vi "Broadcast Status.vi"(8 "error in (no error)":errorcluster, 11 "Actor in":refnum<class "System Status Actor.lvclass">) -> (0 "error out":errorcluster)   [LabVIEW 2020, in "System Status Actor.lvclass"]
uses:
  System Status Actor.lvclass
  System Status Actor.lvclass/System Status Actor.ctl
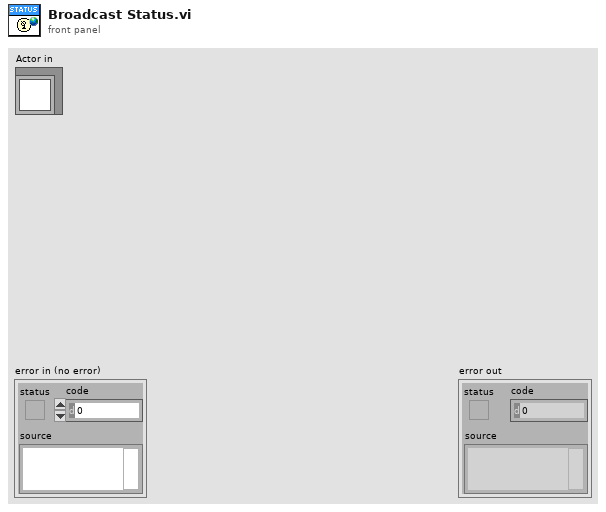
[diagram p1: front panel]
types:
  T1 = typedef "System Status Actor.lvclass/Status.ctl" = cluster{"Memory":cluster{"Total [MB]":dbl, "Used [MB]":dbl, "Free [MB]":dbl}, "Disk":cluster{"Total [MB]":dbl, "Used [MB]":dbl, "Free [MB]":dbl}, "CPU loads":T2[]}
  T2 = typedef "NI_Real-Time Target Support.lvlib/RT CPU Load.ctl" = cluster{"Total (%)":dbl, "Time Critical (%)":dbl, "Timed Structures (%)":dbl, "High (%)":dbl, "Above Normal (%)":dbl, "Normal (%)":dbl, "Background (%)":dbl, "Idle (%)":dbl, "ISR (%)":dbl}
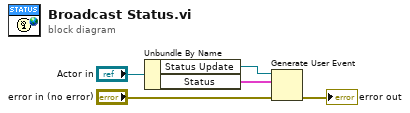
[diagram p0: block diagram]
diagram:
  n1 = Unbundle By Name("Actor in") -> ("Status Update"=w1:refnum<user-event>, "Status"=w4:T1)
  n2 = Generate User Event(user event=w1, event data cluster=w4, error in="error in (no error)") -> (error out=→"error out":errorcluster)  [unwired: 1 in, 1 out]
